vi "Create.vi"(9 "jettl":refnum<class "jettl.lvclass">, 10 "Self Alias":string, 11 "Base Queue in":refnum<class "Base Queue.lvclass">) -> (3 "Base Queue out":refnum<class "Base Queue.lvclass">)   [LabVIEW 2021, in "jettl.lvlib" / "Base Queue.lvlib" / "Base Queue.lvclass"]
uses:
  Base Queue.lvclass
  jettl.lvlib
  Error/Error.lvlib
  Addresses/Addresses.lvlib
  Msg Type Strategy/Msg Type Strategy/Msg Type Strategy.lvclass
  jettl/jettl.lvclass
  C:/git/jettl/jettl/jettl/jettl/jettl.lvclass
  C:/git/jettl/jettl/Merge Error Msg Strategy/Merge Error/Merge Error.lvclass
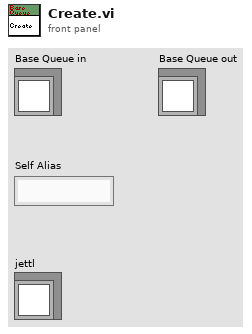
[diagram p1: front panel]
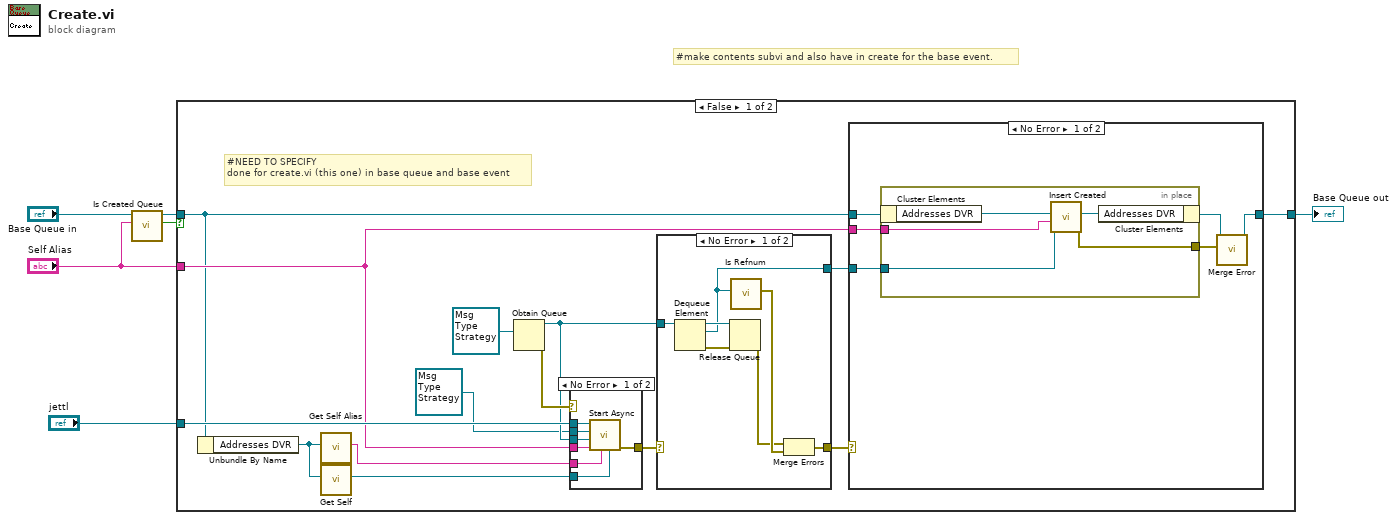
[diagram p0: block diagram]
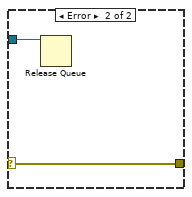
[diagram p2: hidden frame]
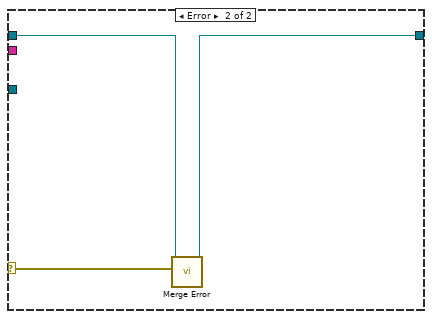
[diagram p4: hidden frame]
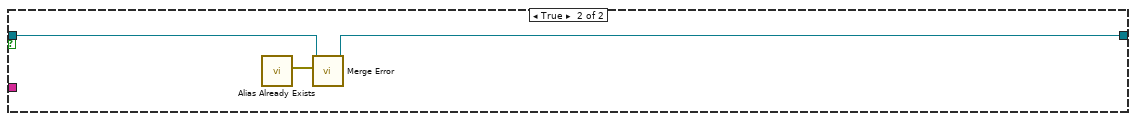
[diagram p5: hidden frame]
diagram:
  # "#make contents subvi and also have in create for the base event."
  n1 = call-dynamic "Is Created Queue.vi"("Created Queue Alias"="Self Alias", "Base Queue in"="Base Queue in") -> ("Is Created Queue?"=w5:bool, "Base Queue out"=w4:refnum<class "Base Queue.lvclass">)  [unwired: 8 in]
  n2 = case shown="False" w5 {
    tunnel: "jettl" -> [w19 _]
    tunnel: w4 -> [w11 w54]
    tunnel: "Self Alias" -> [w18 _]
    tunnel: [w20 w53] -> w6
    frame False {
      # "#NEED TO SPECIFY\ndone for create.vi (this one) in base queue and base event"
      n3 = Unbundle By Name(w11) -> ("Addresses DVR"=w10:refnum<data-value>)
      n4 = call "Get Self Alias.vi"("Addresses DVR"=w10) -> ("Self Alias"=w8:string)  [unwired: 9 in, 1 out]
      n5 = call "Get Self.vi"("Addresses DVR"=w10) -> ("Self"=w9:refnum<class "Msg Type Strategy.lvclass">)  [unwired: 9 in, 1 out]
      n6 = Obtain Queue(element data type=refnum<class "Msg Type Strategy.lvclass"> refnum ("Self")) -> (queue out=w14:refnum<queue>, error out=w17:errorcluster)  [unwired: 4 in, 1 out]
      n7 = case shown="No Error" w17 {
        selector: w17 -> [_ w37]
        tunnel: [w35 w37] -> w15
        tunnel: w19 -> [w36 _]
        tunnel: w14 -> [w31 _]
        tunnel: w18 -> [w32 _]
        tunnel: w9 -> [w34 _]
        tunnel: w8 -> [w33 _]
        tunnel: refnum<class "Msg Type Strategy.lvclass"> refnum ("Msg Type Strategy") -> [w30 _]
        frame No Error {
          n8 = call "Start Async.vi"("Creator"=w34, "Creator Alias"=w33, "Self Alias"=w32, "Queue of Self"=w31, "Msg Type Strategy"=w30, 11:w36) -> ("error out"=w35:errorcluster)  [unwired: 5 in]
        }
        frame Error {
        }
      }
      n9 = case shown="No Error" w15 {
        selector: w15 -> [_ w29]
        tunnel: [w25 w29] -> w16
        tunnel: w14 -> [w22 w28]
        tunnel: [w21 _] -> w13
        frame No Error {
          n10 = Dequeue Element(queue=w22) -> (queue out=w26:refnum<queue>, element=w21:refnum<class "Msg Type Strategy.lvclass">, error out=w27:errorcluster)  [unwired: 2 in, 1 out]
          n11 = Release Queue(queue=w26, error in (no error)=w27) -> (error out=w23:errorcluster)  [unwired: 1 in, 2 out]
          n12 = call "Is Refnum.vi"("Self"=w21) -> ("Error"=w24:errorcluster)  [unwired: 10 in]
          n13 = Merge Errors(w23, w24) -> (w25:errorcluster)
        }
        frame Error {
          n14 = Release Queue(queue=w28) -> ()  [unwired: 2 in, 3 out]
        }
      }
      n15 = case shown="No Error" w16 {
        selector: w16 -> [_ w49]
        tunnel: w11 -> [w40 w51]
        tunnel: [w41 w50] -> w20
        tunnel: w13 -> [w43 _]
        tunnel: w18 -> [w42 _]
        frame No Error {
          n16 = in-place {
            in-place-border: w43 -> [w45]
            in-place-border: w42 -> [w46]
            in-place-border: [w44] -> w38
            n17 = in-place-cluster #1(w40) -> ("Addresses DVR"=w48:refnum<data-value>)
            n18 = call "Insert Created.vi"("Self"=w45, "Self Alias"=w46, "Addresses DVR in"=w48) -> ("error out"=w44:errorcluster, "Addresses DVR out"=w47:refnum<data-value>)  [unwired: 7 in]
            n19 = in-place-cluster #1("Addresses DVR"=w47) -> (w39:refnum<class "Base Queue.lvclass">)
          }
          n20 = call-dynamic "Merge Error.vi"("Error"=w38, "Base Queue in"=w39) -> ("Base Queue out"=w41:refnum<class "Base Queue.lvclass">)  [unwired: 9 in]
        }
        frame Error {
          n21 = call-dynamic "Merge Error.vi"("Error"=w49, "Base Queue in"=w51) -> ("Base Queue out"=w50:refnum<class "Base Queue.lvclass">)  [unwired: 9 in]
        }
      }
    }
    frame True {
      n22 = call "Alias Already Exists.vi"() -> ("Error"=w52:errorcluster)  [unwired: 11 in]
      n23 = call-dynamic "Merge Error.vi"("Error"=w52, "Base Queue in"=w54) -> ("Base Queue out"=w53:refnum<class "Base Queue.lvclass">)  [unwired: 9 in]
    }
  }
  "Base Queue out" <- w6
